vi "real pool auto routine 2.vi"(0 "ROI Descriptor (Geometric Matching 1)":T1={"Global Rectangle"=[20, 20, 1364, 1012], "Contours"=[{"ID"=enum."External", "Type"=3, "Coordinates"=[20, 20, 1364, 1012]}]} {"Contours"."Type" items=["No Selection", "Point", "Line", "Rectangle", "Oval", "Polygon", "Freehand Region", "Annulus", "Unused2", "Unused3", "Broken Line", "Freehand Line", "Rotated Rectangle"]}, 2 "Template File Path (Geometric Matching 1)":path=path "C:/Users/GARLAND/Documents/Projects/Robotics I/Robotics I 3390 2012/Final project/Labview/Real Pool navigation/real pool location templete.png", 3 "ROI Descriptor (Geometric Matching 2)":T1={"Global Rectangle"=[20, 20, 1364, 1012], "Contours"=[{"ID"=enum."External", "Type"=3, "Coordinates"=[20, 20, 1364, 1012]}]} {"Contours"."Type" items=["No Selection", "Point", "Line", "Rectangle", "Oval", "Polygon", "Freehand Region", "Annulus", "Unused2", "Unused3", "Broken Line", "Freehand Line", "Rotated Rectangle"]}, 4 "Settings (Geometric Matching 2)":T4={"Curve Parameters"={"Extraction Mode"=0, "Edge Threshold"=75, "Edge Filter Size"=1, "Min Length"=25, "Row Search Step Size"=15, "Col Search Step Size"=15, "Max Endpoint Gap"=10, "Closed"=FALSE, "Subpixel"=FALSE}, "Match Mode"={"Rotation"=TRUE, "Scale"=FALSE, "Occlusion"=TRUE, "Reserved"=FALSE, "Reserved"=FALSE, "Reserved"=FALSE}, "Range Settings"=[{"Match Constraints"=0, "Min"=0.0, "Max"=360.0}, {"Match Constraints"=2, "Min"=0.0, "Max"=25.0}], "Number of Matches"=1, "Minimum Match Score"=800.0, "SubPixel Accuracy"=FALSE, "Adv. Geometric Match Options 2"=[{"Setup Data Item"=21, "Item Value"=0.0}, {"Setup Data Item"=22, "Item Value"=1.0}]} {"Curve Parameters"."Extraction Mode" items=["Normal", "Uniform Regions"]; "Curve Parameters"."Edge Filter Size" items=["Fine", "Normal", "Contour Tracing"]; "Curve Parameters"."Max Endpoint Gap" min=0; "Curve Parameters"."Col Search Step Size" min=1 max=255 step=1; "Curve Parameters"."Row Search Step Size" min=1 max=255 step=1; "Curve Parameters"."Min Length" min=0; "Curve Parameters"."Edge Threshold" min=1 max=350 step=1; "Range Settings"."Max" format="%.2f"; "Range Settings"."Min" format="%.2f"; "Range Settings"."Match Constraints" items=["Rotation Angle (degrees)", "Scale Factor (%)", "Occlusion (%)"]; "Adv. Geometric Match Options 2"."Setup Data Item" items=["Curve Extraction Mode", "Curve Edge Threshold", "Curve Edge Filter Size", "Min Curve Length", "Curve Row Search Step Size", "Curve Col Search Step Size", "Curve Max Endpoint Gap", "Extract Closed Curves", "Enable Subpixel Curve Extraction", "Enable Correlation Score", "Enable Subpixel Accuracy", "Subpixel Iterations", "Subpixel Tolerance", "Initial Match List Length", "Enable Target Template Curve Score", "Min Match Separation Distance", "Min Match Separation Angle", "Min Match Separation Scale", "Max Match Overlap", "Enable Coarse Result", "Enable Calibration Support", "Enable Contrast Reversal", "Search Strategy", "Refinement Match Factor", "Subpixel Match Factor"]}, 5 "Template File Path (Geometric Matching 2)":path=path "C:/Users/GARLAND/Documents/Projects/Robotics I/Robotics I 3390 2012/Final project/Labview/Real Pool navigation/real pool boat templete.png", 6 "ROI Descriptor (Geometric Matching 3)":T1={"Global Rectangle"=[20, 20, 1364, 1012], "Contours"=[{"ID"=enum."External", "Type"=3, "Coordinates"=[20, 20, 1364, 1012]}]} {"Contours"."Type" items=["No Selection", "Point", "Line", "Rectangle", "Oval", "Polygon", "Freehand Region", "Annulus", "Unused2", "Unused3", "Broken Line", "Freehand Line", "Rotated Rectangle"]}, 7 "error in":errorcluster, 8 "Settings (Geometric Matching 3)":T4={"Curve Parameters"={"Extraction Mode"=0, "Edge Threshold"=75, "Edge Filter Size"=1, "Min Length"=25, "Row Search Step Size"=15, "Col Search Step Size"=15, "Max Endpoint Gap"=10, "Closed"=FALSE, "Subpixel"=FALSE}, "Match Mode"={"Rotation"=TRUE, "Scale"=FALSE, "Occlusion"=TRUE, "Reserved"=FALSE, "Reserved"=FALSE, "Reserved"=FALSE}, "Range Settings"=[{"Match Constraints"=0, "Min"=0.0, "Max"=360.0}, {"Match Constraints"=2, "Min"=0.0, "Max"=25.0}], "Number of Matches"=1, "Minimum Match Score"=800.0, "SubPixel Accuracy"=FALSE, "Adv. Geometric Match Options 2"=[{"Setup Data Item"=21, "Item Value"=0.0}, {"Setup Data Item"=22, "Item Value"=1.0}]} {"Curve Parameters"."Extraction Mode" items=["Normal", "Uniform Regions"]; "Curve Parameters"."Edge Filter Size" items=["Fine", "Normal", "Contour Tracing"]; "Curve Parameters"."Max Endpoint Gap" min=0; "Curve Parameters"."Col Search Step Size" min=1 max=255 step=1; "Curve Parameters"."Row Search Step Size" min=1 max=255 step=1; "Curve Parameters"."Min Length" min=0; "Curve Parameters"."Edge Threshold" min=1 max=350 step=1; "Range Settings"."Max" format="%.2f"; "Range Settings"."Min" format="%.2f"; "Range Settings"."Match Constraints" items=["Rotation Angle (degrees)", "Scale Factor (%)", "Occlusion (%)"]; "Adv. Geometric Match Options 2"."Setup Data Item" items=["Curve Extraction Mode", "Curve Edge Threshold", "Curve Edge Filter Size", "Min Curve Length", "Curve Row Search Step Size", "Curve Col Search Step Size", "Curve Max Endpoint Gap", "Extract Closed Curves", "Enable Subpixel Curve Extraction", "Enable Correlation Score", "Enable Subpixel Accuracy", "Subpixel Iterations", "Subpixel Tolerance", "Initial Match List Length", "Enable Target Template Curve Score", "Min Match Separation Distance", "Min Match Separation Angle", "Min Match Separation Scale", "Max Match Overlap", "Enable Coarse Result", "Enable Calibration Support", "Enable Contrast Reversal", "Search Strategy", "Refinement Match Factor", "Subpixel Match Factor"]}, 9 "Template File Path (Geometric Matching 3)":path=path "C:/Users/GARLAND/Documents/Projects/Robotics I/Robotics I 3390 2012/Final project/Labview/Real Pool navigation/real pool bouy templete.png", 10 "ROI Descriptor (Pattern Matching 1)":T1={"Global Rectangle"=[20, 20, 1364, 1012], "Contours"=[{"ID"=enum."External", "Type"=12, "Coordinates"=[20, 20, 1364, 1012, 0]}]} {"Contours"."Type" items=["No Selection", "Point", "Line", "Rectangle", "Oval", "Polygon", "Freehand Region", "Annulus", "Unused2", "Unused3", "Broken Line", "Freehand Line", "Rotated Rectangle"]}, 17 "Template File Path (Pattern Matching 1)":path=path "C:/Users/GARLAND/Documents/Projects/Robotics I/Robotics I 3390 2012/Final project/Labview/Real Pool navigation/real pool whale templete.png", 18 "ROI Descriptor (Geometric Matching 5)":T1={"Global Rectangle"=[20, 20, 1364, 1012], "Contours"=[{"ID"=enum."External", "Type"=3, "Coordinates"=[20, 20, 1364, 1012]}]} {"Contours"."Type" items=["No Selection", "Point", "Line", "Rectangle", "Oval", "Polygon", "Freehand Region", "Annulus", "Unused2", "Unused3", "Broken Line", "Freehand Line", "Rotated Rectangle"]}, 19 "Settings (Geometric Matching 5)":T4={"Curve Parameters"={"Extraction Mode"=0, "Edge Threshold"=75, "Edge Filter Size"=1, "Min Length"=25, "Row Search Step Size"=15, "Col Search Step Size"=15, "Max Endpoint Gap"=10, "Closed"=FALSE, "Subpixel"=FALSE}, "Match Mode"={"Rotation"=TRUE, "Scale"=FALSE, "Occlusion"=TRUE, "Reserved"=FALSE, "Reserved"=FALSE, "Reserved"=FALSE}, "Range Settings"=[{"Match Constraints"=0, "Min"=0.0, "Max"=360.0}, {"Match Constraints"=2, "Min"=0.0, "Max"=25.0}], "Number of Matches"=1, "Minimum Match Score"=800.0, "SubPixel Accuracy"=FALSE, "Adv. Geometric Match Options 2"=[{"Setup Data Item"=21, "Item Value"=0.0}, {"Setup Data Item"=22, "Item Value"=1.0}]} {"Curve Parameters"."Extraction Mode" items=["Normal", "Uniform Regions"]; "Curve Parameters"."Edge Filter Size" items=["Fine", "Normal", "Contour Tracing"]; "Curve Parameters"."Max Endpoint Gap" min=0; "Curve Parameters"."Col Search Step Size" min=1 max=255 step=1; "Curve Parameters"."Row Search Step Size" min=1 max=255 step=1; "Curve Parameters"."Min Length" min=0; "Curve Parameters"."Edge Threshold" min=1 max=350 step=1; "Range Settings"."Max" format="%.2f"; "Range Settings"."Min" format="%.2f"; "Range Settings"."Match Constraints" items=["Rotation Angle (degrees)", "Scale Factor (%)", "Occlusion (%)"]; "Adv. Geometric Match Options 2"."Setup Data Item" items=["Curve Extraction Mode", "Curve Edge Threshold", "Curve Edge Filter Size", "Min Curve Length", "Curve Row Search Step Size", "Curve Col Search Step Size", "Curve Max Endpoint Gap", "Extract Closed Curves", "Enable Subpixel Curve Extraction", "Enable Correlation Score", "Enable Subpixel Accuracy", "Subpixel Iterations", "Subpixel Tolerance", "Initial Match List Length", "Enable Target Template Curve Score", "Min Match Separation Distance", "Min Match Separation Angle", "Min Match Separation Scale", "Max Match Overlap", "Enable Coarse Result", "Enable Calibration Support", "Enable Contrast Reversal", "Search Strategy", "Refinement Match Factor", "Subpixel Match Factor"]}, 21 "Template File Path (Geometric Matching 5)":path=path "C:/Users/GARLAND/Documents/Projects/Robotics I/Robotics I 3390 2012/Final project/Labview/Real Pool navigation/real pool square templete.png", 22 "ROI Descriptor (Geometric Matching 6)":T1={"Global Rectangle"=[20, 20, 1364, 1012], "Contours"=[{"ID"=enum."External", "Type"=3, "Coordinates"=[20, 20, 1364, 1012]}]} {"Contours"."Type" items=["No Selection", "Point", "Line", "Rectangle", "Oval", "Polygon", "Freehand Region", "Annulus", "Unused2", "Unused3", "Broken Line", "Freehand Line", "Rotated Rectangle"]}) -> (20 "Matches (Geometric Matching 1)":T6[](array[typedef]) {"Correlation Score" format="%.2f"; "Target Template Curve Score" format="%.2f"; "Template Target Curve Score" format="%.2f"; "Bounding Box"."y" format="%.2f"; "Bounding Box"."x" format="%.2f"; "Position"."y" format="%.2f"; "Position"."x" format="%.2f"; "Score" format="%.2f"; "Scale" format="%.2f"; "Angle" format="%.2f"; "Occlusion %" format="%.2f"}, 23 "Matches (Geometric Matching 2)":T6[](array[typedef]) {"Correlation Score" format="%.2f"; "Target Template Curve Score" format="%.2f"; "Template Target Curve Score" format="%.2f"; "Bounding Box"."y" format="%.2f"; "Bounding Box"."x" format="%.2f"; "Position"."y" format="%.2f"; "Position"."x" format="%.2f"; "Score" format="%.2f"; "Scale" format="%.2f"; "Angle" format="%.2f"; "Occlusion %" format="%.2f"}, 24 "Matches (Geometric Matching 3)":T6[](array[typedef]) {"Correlation Score" format="%.2f"; "Target Template Curve Score" format="%.2f"; "Template Target Curve Score" format="%.2f"; "Bounding Box"."y" format="%.2f"; "Bounding Box"."x" format="%.2f"; "Position"."y" format="%.2f"; "Position"."x" format="%.2f"; "Score" format="%.2f"; "Scale" format="%.2f"; "Angle" format="%.2f"; "Occlusion %" format="%.2f"}, 25 "Matches (Pattern Matching 1)":T7(array[cluster]) {"Bounding Box"."y" format="%.2f"; "Bounding Box"."x" format="%.2f"; "Position"."y" format="%.2f"; "Position"."x" format="%.2f"; "Score" format="%.2f"; "Scale" format="%.2f"; "Angle" format="%.2f"}, 26 "Matches (Geometric Matching 5)":T6[](array[typedef]) {"Correlation Score" format="%.2f"; "Target Template Curve Score" format="%.2f"; "Template Target Curve Score" format="%.2f"; "Bounding Box"."y" format="%.2f"; "Bounding Box"."x" format="%.2f"; "Position"."y" format="%.2f"; "Position"."x" format="%.2f"; "Score" format="%.2f"; "Scale" format="%.2f"; "Angle" format="%.2f"; "Occlusion %" format="%.2f"}, 27 "error out":errorcluster)   [LabVIEW 2011]
uses:
  <vilib>/vision/Pattern Matching.llb/IMAQ GM Match Report.ctl
  <vilib>/vision/Pattern Matching.llb/IMAQ Curve Parameters.ctl
  <vilib>/vision/Pattern Matching.llb/IMAQ Match Range Setting.ctl
panel:
  out "Image Out":T5(plugin-control)
  # "Range"
  # "Range"
  # "Range"
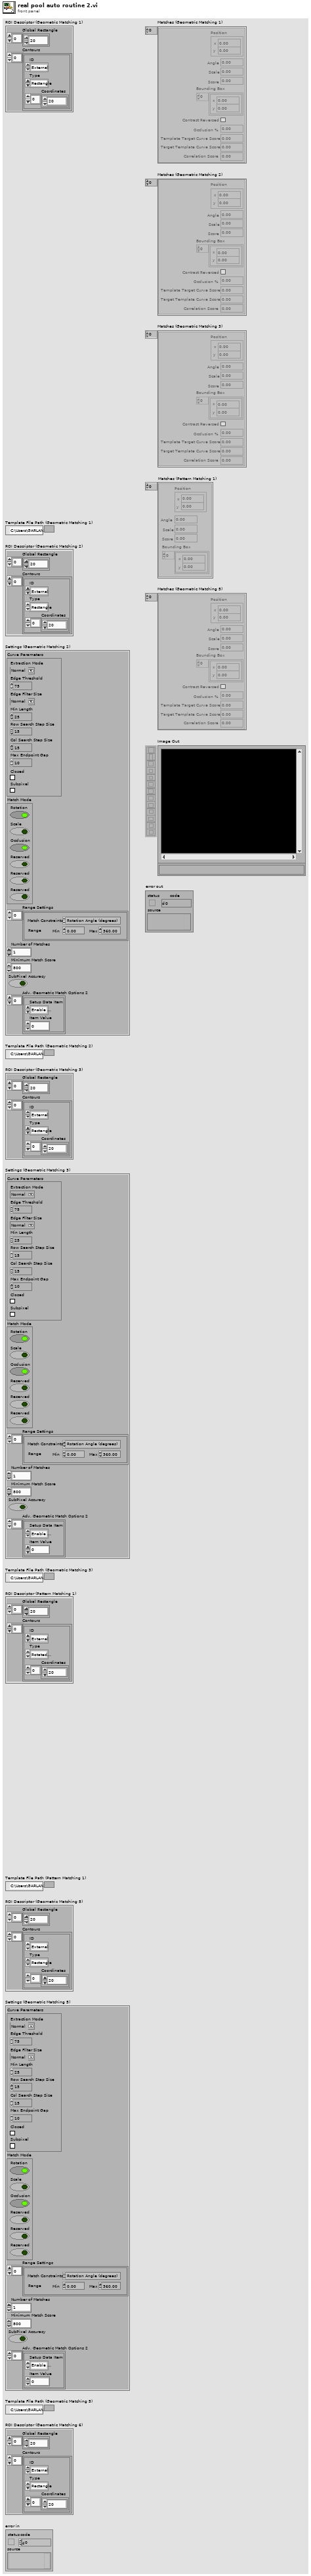
[diagram p1: front panel]
types:
  T1 = cluster{"Global Rectangle":i32[], "Contours":cluster{"ID":enum32{"External", "Internal"}, "Type":u32, "Coordinates":i32[]}[]}
  T2 = typedef "IMAQ Curve Parameters.ctl" = cluster{"Extraction Mode":u32, "Edge Threshold":i32, "Edge Filter Size":u32, "Min Length":i32, "Row Search Step Size":i32, "Col Search Step Size":i32, "Max Endpoint Gap":i32, "Closed":bool, "Subpixel":bool}
  T3 = typedef "IMAQ Match Range Setting.ctl" = cluster{"Match Constraints":u32, "Min":dbl, "Max":dbl}
  T4 = cluster{"Curve Parameters":T2, "Match Mode":cluster{"Rotation":bool, "Scale":bool, "Occlusion":bool, "Reserved":bool, "Reserved":bool, "Reserved":bool}, "Range Settings":T3[], "Number of Matches":i32, "Minimum Match Score":sgl, "SubPixel Accuracy":bool, "Adv. Geometric Match Options 2":cluster{"Setup Data Item":u16, "Item Value":dbl}[]}
  T5 = typedef "IMAQ Image.ctl" = refnum<image>
  T6 = typedef "IMAQ GM Match Report.ctl" = cluster{"Position":cluster{"x":sgl, "y":sgl}, "Angle":sgl, "Scale":sgl, "Score":sgl, "Bounding Box":cluster{"x":sgl, "y":sgl}[], "Contrast Reversed":bool, "Occlusion %":sgl, "Template Target Curve Score":sgl, "Target Template Curve Score":sgl, "Correlation Score":sgl}
  T7 = cluster{"Position":cluster{"x":sgl, "y":sgl}, "Angle":sgl, "Scale":sgl, "Score":sgl, "Bounding Box":cluster{"x":sgl, "y":sgl}[]}[]
  T8 = typedef "Image Type" = u32
  T9 = cluster{"Match Mode (Pattern Matching 1)":u16, "Subpixel Accuracy (Pattern Matching 1)":bool, "Rotation Angle Ranges (degrees) (Pattern Matching 1)":cluster{sgl, sgl}[]}
  T10 = cluster{"ROI Descriptor (Pattern Matching 1)":cluster{"Global Rectangle":i32[], "Contours":cluster{"ID":enum32{"External", "Internal"}, "Type":u32, "Coordinates":i32[]}[]}, "Number of Matches Requested (Pattern Matching 1)":i32, "Minimum Match Score (Pattern Matching 1)":sgl}
diagram:
  w41 = u16 0 items=["Shift Invariant", "Rotation Invariant"] ("Match Mode (Pattern Matching 1)")
  w2 = u32 0 items=["Grayscale", "Binary", "Gradient", "Rainbow", "Temperature", "User Defined"] ("Palette")
  w5 = T4 {"Curve Parameters"={"Extraction Mode"=0, "Edge Threshold"=75, "Edge Filter Size"=1, "Min Length"=25, "Row Search Step Size"=15, "Col Search Step Size"=15, "Max Endpoint Gap"=10, "Closed"=FALSE, "Subpixel"=FALSE}, "Match Mode"={"Rotation"=TRUE, "Scale"=FALSE, "Occlusion"=TRUE, "Reserved"=FALSE, "Reserved"=FALSE, "Reserved"=FALSE}, "Range Settings"=[{"Match Constraints"=0, "Min"=0.0, "Max"=360.0}, {"Match Constraints"=2, "Min"=0.0, "Max"=25.0}], "Number of Matches"=1, "Minimum Match Score"=800.0, "SubPixel Accuracy"=FALSE, "Adv. Geometric Match Options 2"=[{"Setup Data Item"=21, "Item Value"=0.0}, {"Setup Data Item"=22, "Item Value"=1.0}]}  # Settings
  w4 = "Geometric Matching 6" ("Step Name")
  w15 = "Geometric Matching 5" ("Step Name")
  w27 = "Pattern Matching 1" ("Step Name")
  w43 = "Geometric Matching 3" ("Step Name")
  w54 = "Geometric Matching 2" ("Step Name")
  w65 = "Geometric Matching 1" ("Step Name")
  w76 = T8 0 items=["Grayscale (U8)", "Grayscale (I16)", "Grayscale (SGL)", "Complex (CSG)", "RGB (U32)", "HSL (U32)", "RGB (U64)", "Grayscale (U16)"] ("Image Type")
  # "Geometric Matching"
  # "Geometric Matching"
  # "Pattern Matching"
  # "Geometric Matching"
  # "Geometric Matching"
  # "Geometric Matching"
  n1 = Call Chain() -> (call chain=w80:string[])
  n2 = Index Array(array=w80) -> (element=w79:string)  [unwired: 1 in]
  n3 = call "File Dialog"("prompt"="Select an image file...") -> ("selected path"=w77:path)  [unwired: 6 in, 8 out]
  n4 = call "IMAQ Create"("Image Name"=w79, "Image Type"=w76, "error in (no error)"="error in") -> ("New Image"=w83:T5, "error out"=w82:errorcluster)  [unwired: 1 in, 1 out]
  n5 = call "IMAQ ReadFile"("File Path"=w77, "error in (no error)"=w82, "Image"=w83) -> ("error out"=w84:errorcluster, "Image Out"=w73:T5)  [unwired: 2 in, 5 out]
  n6 = Unbundle By Name(w84) -> ("code"=w68:i32)
  n7 = case shown="Default" w68 {
    tunnel: "Template File Path (Geometric Matching 1)" -> [_ w90]
    tunnel: w84 -> [_ w89]
    tunnel: T4 {"Curve Parameters"={"Extraction Mode"=0, "Edge Threshold"=75, "Edge Filter Size"=1, "Min Length"=25, "Row Search Step Size"=15, "Col Search Step Size"=15, "Max Endpoint Gap"=10, "Closed"=FALSE, "Subpixel"=FALSE}, "Match Mode"={"Rotation"=TRUE, "Scale"=FALSE, "Occlusion"=TRUE, "Reserved"=FALSE, "Reserved"=FALSE, "Reserved"=FALSE}, "Range Settings"=[{"Match Constraints"=0, "Min"=0.0, "Max"=360.0}, {"Match Constraints"=2, "Min"=0.0, "Max"=25.0}], "Number of Matches"=1, "Minimum Match Score"=800.0, "SubPixel Accuracy"=FALSE, "Adv. Geometric Match Options 2"=[{"Setup Data Item"=21, "Item Value"=0.0}, {"Setup Data Item"=22, "Item Value"=1.0}]} ("Settings (Geometric Matching 1)") -> [_ w97]
    tunnel: "ROI Descriptor (Geometric Matching 1)" -> [_ w96]
    tunnel: w73 -> [w85 w91]
    tunnel: [_ w95] -> w72
    tunnel: [_ w94] -> w70
    tunnel: [_ w93] -> w69
    tunnel: [_ w92] -> _
    tunnel: [w85 w91] -> w67
    tunnel: w65 -> [_ w86]
    frame -1074396199, -1074396198 {
      # "Discard Coordinate System Error"
    }
    frame Default {
      n8 = while {
        shift-right: [w106] -> w87
        shift-left: _ -> [w105]
        tunnel: [w103] -> w88
        tunnel: w89 -> [w102]
        tunnel: w90 -> [w98]
        tunnel: w86 -> [w101]
        shift-right: [w98] -> _
        shift-left: _ -> [w100]
        stop <- FALSE continue-if-true
        n9 = Not Equal?(x=w100, y=w98) -> (x != y?=w99:bool)
        n10 = case shown="True" w99 {
          tunnel: [w108 w120] -> w106
          tunnel: w105 -> [w108 w112]
          tunnel: [w107 w117] -> w103
          tunnel: w102 -> [w107 w113]
          tunnel: w101 -> [_ w114]
          tunnel: w98 -> [_ w110]
          frame False {
          }
          frame True {
            n11 = Call Chain() -> (call chain=w116:string[])
            n12 = stacked-sequence {
              tunnel: w113 -> [w124]
              tunnel: w112 -> [w123]
              tunnel: [w124] -> w111
              frame #0 {
                n13 = call "IMAQ Dispose"("Image"=w123) -> ()  [unwired: 2 in, 4 out]
              }
            }
            n14 = Index Array(array=w116) -> (element=w115:string)  [unwired: 1 in]
            n15 = Format Into String(format string="GM Template %s %s" ("Image Name"), w115, w114) -> (resulting string=w122:string)  [unwired: 2 in, 1 out]
            n16 = call "IMAQ Create"("Image Name"=w122, "error in (no error)"=w111) -> ("New Image"=w119:T5, "error out"=w118:errorcluster)  [unwired: 2 in, 1 out]
            n17 = call <vilib>:"IVA Get Alternate Path.vi"("Path In"=w110) -> ("Path Out"=w109:path)  [unwired: 10 out]
            n18 = call "IMAQ Read Image And Vision Info"("File Path"=w109, "error in (no error)"=w118, "Image"=w119) -> ("error out"=w117:errorcluster, "Image Out"=w120:T5)  [unwired: 1 in, 6 out]
          }
        }
      }
      n19 = call <vilib>:"IVA Match Geometric Pattern Algorithm 2.vi"("Template"=w87, "error in (no error)"=w88, "Settings"=w97, "ROI Descriptor"=w96, "Image"=w91) -> ("error out"=w95:errorcluster, "Calibrated Matches"=w93:T6[], "Matches"=w94:T6[], "Number of Matches"=w92:i32)  [unwired: 1 in, 2 out]
    }
  }
  "Matches (Geometric Matching 1)" <- w70
  n20 = call <vilib>:"IVA Store Match Geometric Pattern Results.vi"("Calibrated Matches"=w69, "error in (no error)"=w72, "Matches"=w70, "Step Name"=w65, "Image in"=w67) -> ("error out"=w71:errorcluster, "Image dup"=w62:T5)  [unwired: 5 out]
  n21 = Unbundle By Name(w71) -> ("code"=w57:i32)
  n22 = case shown="Default" w57 {
    tunnel: "Template File Path (Geometric Matching 2)" -> [_ w127]
    tunnel: w71 -> [_ w128]
    tunnel: "Settings (Geometric Matching 2)" -> [_ w137]
    tunnel: "ROI Descriptor (Geometric Matching 2)" -> [_ w136]
    tunnel: w62 -> [w125 w131]
    tunnel: [_ w135] -> w61
    tunnel: [_ w134] -> w59
    tunnel: [_ w133] -> w58
    tunnel: [_ w132] -> _
    tunnel: [w125 w131] -> w56
    tunnel: w54 -> [_ w126]
    frame -1074396199, -1074396198 {
      # "Discard Coordinate System Error"
    }
    frame Default {
      n23 = while {
        shift-right: [w146] -> w129
        shift-left: _ -> [w145]
        tunnel: [w143] -> w130
        tunnel: w128 -> [w142]
        tunnel: w127 -> [w138]
        tunnel: w126 -> [w141]
        shift-right: [w138] -> _
        shift-left: _ -> [w140]
        stop <- FALSE continue-if-true
        n24 = Not Equal?(x=w140, y=w138) -> (x != y?=w139:bool)
        n25 = case shown="True" w139 {
          tunnel: [w148 w160] -> w146
          tunnel: w145 -> [w148 w152]
          tunnel: [w147 w157] -> w143
          tunnel: w142 -> [w147 w153]
          tunnel: w141 -> [_ w154]
          tunnel: w138 -> [_ w150]
          frame False {
          }
          frame True {
            n26 = Call Chain() -> (call chain=w156:string[])
            n27 = stacked-sequence {
              tunnel: w153 -> [w164]
              tunnel: w152 -> [w163]
              tunnel: [w164] -> w151
              frame #0 {
                n28 = call "IMAQ Dispose"("Image"=w163) -> ()  [unwired: 2 in, 4 out]
              }
            }
            n29 = Index Array(array=w156) -> (element=w155:string)  [unwired: 1 in]
            n30 = Format Into String(format string="GM2 Template %s %s" ("Image Name"), w155, w154) -> (resulting string=w162:string)  [unwired: 2 in, 1 out]
            n31 = call "IMAQ Create"("Image Name"=w162, "error in (no error)"=w151) -> ("New Image"=w159:T5, "error out"=w158:errorcluster)  [unwired: 2 in, 1 out]
            n32 = call <vilib>:"IVA Get Alternate Path.vi"("Path In"=w150) -> ("Path Out"=w149:path)  [unwired: 10 out]
            n33 = call "IMAQ Read Image And Vision Info"("File Path"=w149, "error in (no error)"=w158, "Image"=w159) -> ("error out"=w157:errorcluster, "Image Out"=w160:T5)  [unwired: 1 in, 6 out]
          }
        }
      }
      n34 = call <vilib>:"IVA Match Geometric Pattern Algorithm 3.vi"("Template"=w129, "error in (no error)"=w130, "Settings"=w137, "ROI Descriptor"=w136, "Image"=w131) -> ("error out"=w135:errorcluster, "Calibrated Matches"=w133:T6[], "Matches"=w134:T6[], "Number of Matches"=w132:i32)  [unwired: 3 out]
    }
  }
  "Matches (Geometric Matching 2)" <- w59
  n35 = call <vilib>:"IVA Store Match Geometric Pattern Results.vi"("Calibrated Matches"=w58, "error in (no error)"=w61, "Matches"=w59, "Step Name"=w54, "Image in"=w56) -> ("error out"=w60:errorcluster, "Image dup"=w51:T5)  [unwired: 5 out]
  n36 = Unbundle By Name(w60) -> ("code"=w46:i32)
  n37 = case shown="Default" w46 {
    tunnel: "Template File Path (Geometric Matching 3)" -> [_ w167]
    tunnel: w60 -> [_ w168]
    tunnel: "Settings (Geometric Matching 3)" -> [_ w177]
    tunnel: "ROI Descriptor (Geometric Matching 3)" -> [_ w176]
    tunnel: w51 -> [w165 w171]
    tunnel: [_ w175] -> w50
    tunnel: [_ w174] -> w48
    tunnel: [_ w173] -> w47
    tunnel: [_ w172] -> _
    tunnel: [w165 w171] -> w45
    tunnel: w43 -> [_ w166]
    frame -1074396199, -1074396198 {
      # "Discard Coordinate System Error"
    }
    frame Default {
      n38 = while {
        shift-right: [w186] -> w169
        shift-left: _ -> [w185]
        tunnel: [w183] -> w170
        tunnel: w168 -> [w182]
        tunnel: w167 -> [w178]
        tunnel: w166 -> [w181]
        shift-right: [w178] -> _
        shift-left: _ -> [w180]
        stop <- FALSE continue-if-true
        n39 = Not Equal?(x=w180, y=w178) -> (x != y?=w179:bool)
        n40 = case shown="True" w179 {
          tunnel: [w188 w200] -> w186
          tunnel: w185 -> [w188 w192]
          tunnel: [w187 w197] -> w183
          tunnel: w182 -> [w187 w193]
          tunnel: w181 -> [_ w194]
          tunnel: w178 -> [_ w190]
          frame False {
          }
          frame True {
            n41 = Call Chain() -> (call chain=w196:string[])
            n42 = stacked-sequence {
              tunnel: w193 -> [w204]
              tunnel: w192 -> [w203]
              tunnel: [w204] -> w191
              frame #0 {
                n43 = call "IMAQ Dispose"("Image"=w203) -> ()  [unwired: 2 in, 4 out]
              }
            }
            n44 = Index Array(array=w196) -> (element=w195:string)  [unwired: 1 in]
            n45 = Format Into String(format string="GM2 Template %s %s" ("Image Name"), w195, w194) -> (resulting string=w202:string)  [unwired: 2 in, 1 out]
            n46 = call "IMAQ Create"("Image Name"=w202, "error in (no error)"=w191) -> ("New Image"=w199:T5, "error out"=w198:errorcluster)  [unwired: 2 in, 1 out]
            n47 = call <vilib>:"IVA Get Alternate Path.vi"("Path In"=w190) -> ("Path Out"=w189:path)  [unwired: 10 out]
            n48 = call "IMAQ Read Image And Vision Info"("File Path"=w189, "error in (no error)"=w198, "Image"=w199) -> ("error out"=w197:errorcluster, "Image Out"=w200:T5)  [unwired: 1 in, 6 out]
          }
        }
      }
      n49 = call <vilib>:"IVA Match Geometric Pattern Algorithm 3.vi"("Template"=w169, "error in (no error)"=w170, "Settings"=w177, "ROI Descriptor"=w176, "Image"=w171) -> ("error out"=w175:errorcluster, "Calibrated Matches"=w173:T6[], "Matches"=w174:T6[], "Number of Matches"=w172:i32)  [unwired: 3 out]
    }
  }
  "Matches (Geometric Matching 3)" <- w48
  n50 = call <vilib>:"IVA Store Match Geometric Pattern Results.vi"("Calibrated Matches"=w47, "error in (no error)"=w50, "Matches"=w48, "Step Name"=w43, "Image in"=w45) -> ("error out"=w49:errorcluster, "Image dup"=w33:T5)  [unwired: 5 out]
  n51 = Bundle("Match Mode (Pattern Matching 1)"=w41, "Subpixel Accuracy (Pattern Matching 1)"=FALSE, "Rotation Angle Ranges (degrees) (Pattern Matching 1)"=cluster{sgl, sgl}[] [{-20.0, 20.0}]) -> (w38:T9)  [unwired: 1 out]
  n52 = Bundle("ROI Descriptor (Pattern Matching 1)"="ROI Descriptor (Pattern Matching 1)", "Number of Matches Requested (Pattern Matching 1)"=1, "Minimum Match Score (Pattern Matching 1)"=sgl 800.0) -> (w35:T10)  [unwired: 1 out]
  n53 = Unbundle By Name(w49) -> ("code"=w28:i32)
  n54 = case shown="Default" w28 {
    tunnel: "Template File Path (Pattern Matching 1)" -> [_ w210]
    tunnel: w49 -> [_ w209]
    tunnel: [_ w217] -> _
    tunnel: w38 -> [_ w216]
    tunnel: w35 -> [_ w215]
    tunnel: cluster{"X":sgl, "Y":sgl} {"X"=0.0, "Y"=0.0} ("Match Offset (Pattern Matching 1)") -> [_ w214]
    tunnel: w33 -> [w205 w211]
    tunnel: [_ w213] -> w32
    tunnel: [_ w212] -> w30
    tunnel: [w205 w211] -> w29
    tunnel: w27 -> [_ w206]
    frame -1074396199, -1074396198 {
      # "Discard\nCoordinate\nSystem Error"
    }
    frame Default {
      n55 = while {
        shift-right: [w226] -> w207
        shift-left: _ -> [w225]
        tunnel: [w223] -> w208
        tunnel: w209 -> [w222]
        tunnel: w210 -> [w219]
        tunnel: w206 -> [w221]
        shift-right: [w219] -> _
        shift-left: _ -> [w220]
        stop <- FALSE continue-if-true
        n56 = Not Equal?(x=w220, y=w219) -> (x != y?=w218:bool)
        n57 = case shown="True" w218 {
          tunnel: [w228 w240] -> w226
          tunnel: w225 -> [w228 w231]
          tunnel: [w227 w237] -> w223
          tunnel: w222 -> [w227 w230]
          tunnel: w219 -> [_ w233]
          tunnel: w221 -> [_ w234]
          frame False {
          }
          frame True {
            n58 = Call Chain() -> (call chain=w236:string[])
            n59 = stacked-sequence {
              tunnel: w231 -> [w244]
              tunnel: w230 -> [w243]
              tunnel: [w243] -> w229
              frame #0 {
                n60 = call "IMAQ Dispose"("Image"=w244) -> ()  [unwired: 2 in, 4 out]
              }
            }
            n61 = Index Array(array=w236) -> (element=w235:string)  [unwired: 1 in]
            n62 = Format Into String(format string="PM Template %s %s" ("Image Name"), w235, w234) -> (resulting string=w242:string)  [unwired: 2 in, 1 out]
            n63 = call "IMAQ Create"("Image Name"=w242, "error in (no error)"=w229) -> ("New Image"=w239:T5, "error out"=w238:errorcluster)  [unwired: 2 in, 1 out]
            n64 = call <vilib>:"IVA Get Alternate Path.vi"("Path In"=w233) -> ("Path Out"=w232:path)  [unwired: 10 out]
            n65 = call "IMAQ Read Image And Vision Info"("File Path"=w232, "error in (no error)"=w238, "Image"=w239) -> ("error out"=w237:errorcluster, "Image Out"=w240:T5)  [unwired: 1 in, 6 out]
          }
        }
      }
      n66 = call <vilib>:"IVA Match Pattern Algorithm 3.vi"("Match Offset"=w214, "Image Template"=w207, "error in (no error)"=w208, "Match Parameters"=w215, "Setup Match Parameters"=w216, "Image"=w211) -> ("error out"=w213:errorcluster, "Number of Matches"=w217:i32, "Matches"=w212:T7)  [unwired: 3 out]
    }
  }
  "Matches (Pattern Matching 1)" <- w30
  n67 = call <vilib>:"IVA Store Match Pattern Results.vi"("error in (no error)"=w32, "Matches"=w30, "Step Name"=w27, "Image in"=w29) -> ("error out"=w31:errorcluster, "Image dup"=w23:T5)  [unwired: 6 out]
  n68 = Unbundle By Name(w31) -> ("code"=w18:i32)
  n69 = case shown="Default" w18 {
    tunnel: "Template File Path (Geometric Matching 5)" -> [_ w247]
    tunnel: w31 -> [_ w248]
    tunnel: "Settings (Geometric Matching 5)" -> [_ w257]
    tunnel: "ROI Descriptor (Geometric Matching 5)" -> [_ w256]
    tunnel: w23 -> [w245 w251]
    tunnel: [_ w255] -> w22
    tunnel: [_ w254] -> w20
    tunnel: [_ w253] -> w19
    tunnel: [_ w252] -> _
    tunnel: [w245 w251] -> w17
    tunnel: w15 -> [_ w246]
    frame -1074396199, -1074396198 {
      # "Discard Coordinate System Error"
    }
    frame Default {
      n70 = while {
        shift-right: [w266] -> w249
        shift-left: _ -> [w265]
        tunnel: [w263] -> w250
        tunnel: w248 -> [w262]
        tunnel: w247 -> [w258]
        tunnel: w246 -> [w261]
        shift-right: [w258] -> _
        shift-left: _ -> [w260]
        stop <- FALSE continue-if-true
        n71 = Not Equal?(x=w260, y=w258) -> (x != y?=w259:bool)
        n72 = case shown="True" w259 {
          tunnel: [w268 w280] -> w266
          tunnel: w265 -> [w268 w272]
          tunnel: [w267 w277] -> w263
          tunnel: w262 -> [w267 w273]
          tunnel: w261 -> [_ w274]
          tunnel: w258 -> [_ w270]
          frame False {
          }
          frame True {
            n73 = Call Chain() -> (call chain=w276:string[])
            n74 = stacked-sequence {
              tunnel: w273 -> [w284]
              tunnel: w272 -> [w283]
              tunnel: [w284] -> w271
              frame #0 {
                n75 = call "IMAQ Dispose"("Image"=w283) -> ()  [unwired: 2 in, 4 out]
              }
            }
            n76 = Index Array(array=w276) -> (element=w275:string)  [unwired: 1 in]
            n77 = Format Into String(format string="GM2 Template %s %s" ("Image Name"), w275, w274) -> (resulting string=w282:string)  [unwired: 2 in, 1 out]
            n78 = call "IMAQ Create"("Image Name"=w282, "error in (no error)"=w271) -> ("New Image"=w279:T5, "error out"=w278:errorcluster)  [unwired: 2 in, 1 out]
            n79 = call <vilib>:"IVA Get Alternate Path.vi"("Path In"=w270) -> ("Path Out"=w269:path)  [unwired: 10 out]
            n80 = call "IMAQ Read Image And Vision Info"("File Path"=w269, "error in (no error)"=w278, "Image"=w279) -> ("error out"=w277:errorcluster, "Image Out"=w280:T5)  [unwired: 1 in, 6 out]
          }
        }
      }
      n81 = call <vilib>:"IVA Match Geometric Pattern Algorithm 3.vi"("Template"=w249, "error in (no error)"=w250, "Settings"=w257, "ROI Descriptor"=w256, "Image"=w251) -> ("error out"=w255:errorcluster, "Calibrated Matches"=w253:T6[], "Matches"=w254:T6[], "Number of Matches"=w252:i32)  [unwired: 3 out]
    }
  }
  "Matches (Geometric Matching 5)" <- w20
  n82 = call <vilib>:"IVA Store Match Geometric Pattern Results.vi"("Calibrated Matches"=w19, "error in (no error)"=w22, "Matches"=w20, "Step Name"=w15, "Image in"=w17) -> ("error out"=w21:errorcluster, "Image dup"=w12:T5)  [unwired: 5 out]
  n83 = Unbundle By Name(w21) -> ("code"=w7:i32)
  n84 = case shown="Default" w7 {
    tunnel: path "C:/Users/GARLAND/Documents/Projects/Robotics I/Robotics I 3390 2012/Final project/Labview/Real Pool navigation/real pool big boat templete.png" ("Template File Path") -> [_ w287]
    tunnel: w21 -> [_ w288]
    tunnel: w5 -> [_ w297]
    tunnel: "ROI Descriptor (Geometric Matching 6)" -> [_ w296]
    tunnel: w12 -> [w285 w291]
    tunnel: [_ w295] -> w11
    tunnel: [_ w294] -> w9
    tunnel: [_ w293] -> w8
    tunnel: [_ w292] -> _
    tunnel: [w285 w291] -> w6
    tunnel: w4 -> [_ w286]
    frame -1074396199, -1074396198 {
      # "Discard Coordinate System Error"
    }
    frame Default {
      n85 = while {
        shift-right: [w306] -> w289
        shift-left: _ -> [w305]
        tunnel: [w303] -> w290
        tunnel: w288 -> [w302]
        tunnel: w287 -> [w298]
        tunnel: w286 -> [w301]
        shift-right: [w298] -> _
        shift-left: _ -> [w300]
        stop <- FALSE continue-if-true
        n86 = Not Equal?(x=w300, y=w298) -> (x != y?=w299:bool)
        n87 = case shown="True" w299 {
          tunnel: [w308 w320] -> w306
          tunnel: w305 -> [w308 w312]
          tunnel: [w307 w317] -> w303
          tunnel: w302 -> [w307 w313]
          tunnel: w301 -> [_ w314]
          tunnel: w298 -> [_ w310]
          frame False {
          }
          frame True {
            n88 = Call Chain() -> (call chain=w316:string[])
            n89 = stacked-sequence {
              tunnel: w313 -> [w324]
              tunnel: w312 -> [w323]
              tunnel: [w324] -> w311
              frame #0 {
                n90 = call "IMAQ Dispose"("Image"=w323) -> ()  [unwired: 2 in, 4 out]
              }
            }
            n91 = Index Array(array=w316) -> (element=w315:string)  [unwired: 1 in]
            n92 = Format Into String(format string="GM2 Template %s %s" ("Image Name"), w315, w314) -> (resulting string=w322:string)  [unwired: 2 in, 1 out]
            n93 = call "IMAQ Create"("Image Name"=w322, "error in (no error)"=w311) -> ("New Image"=w319:T5, "error out"=w318:errorcluster)  [unwired: 2 in, 1 out]
            n94 = call <vilib>:"IVA Get Alternate Path.vi"("Path In"=w310) -> ("Path Out"=w309:path)  [unwired: 10 out]
            n95 = call "IMAQ Read Image And Vision Info"("File Path"=w309, "error in (no error)"=w318, "Image"=w319) -> ("error out"=w317:errorcluster, "Image Out"=w320:T5)  [unwired: 1 in, 6 out]
          }
        }
      }
      n96 = call <vilib>:"IVA Match Geometric Pattern Algorithm 3.vi"("Template"=w289, "error in (no error)"=w290, "Settings"=w297, "ROI Descriptor"=w296, "Image"=w291) -> ("error out"=w295:errorcluster, "Calibrated Matches"=w293:T6[], "Matches"=w294:T6[], "Number of Matches"=w292:i32)  [unwired: 3 out]
    }
  }
  n97 = call <vilib>:"IVA Store Match Geometric Pattern Results.vi"("Calibrated Matches"=w8, "error in (no error)"=w11, "Matches"=w9, "Step Name"=w4, "Image in"=w6) -> ("error out"=w10:errorcluster, "Image dup"=→"Image Out":T5)  [unwired: 5 out]
  n98 = property on="Image Out" class="ImageControl"(error in=w10, "Palette:Palette Type"=w2) -> (error out=→"error out":errorcluster)  [unwired: 1 in, 1 out]
